vi "Open Playback Panel.vi"(9 "Offset":cluster{"dX":i32, "dY":i32}={"dX"=60, "dY"=60}, 10 "DB VI Ref":refnum<vi>, 11 "Playback in":refnum<vi>) -> (3 "Playback out":refnum<vi>)   [LabVIEW 2020]
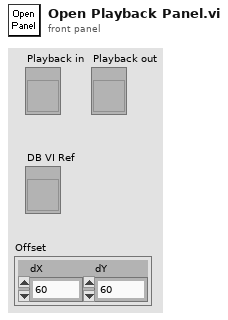
[diagram p1: front panel]
types:
  T1 = typedef "LVRectTypeDef.ctl" = cluster{"Left":i16, "Top":i16, "Right":i16, "Bottom":i16}
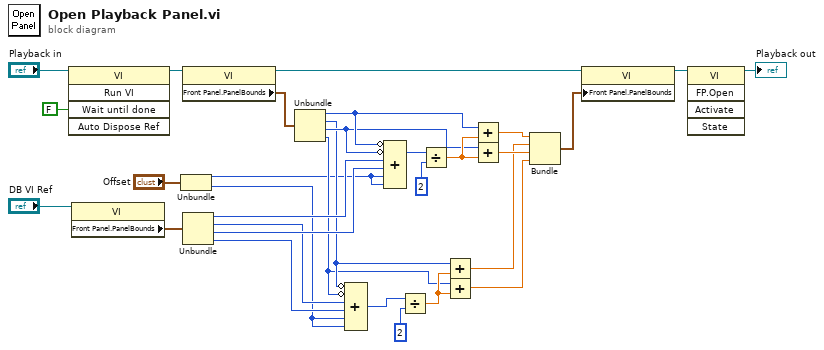
[diagram p0: block diagram]
diagram:
  n1 = invoke class="VI" method="Run VI"(reference="Playback in", "Wait until done"=FALSE ("Wait Until Done")) -> (reference out=w27:refnum<vi>)  [unwired: 3 in, 4 out]
  n2 = property class="VI"(reference="DB VI Ref") -> ("Front Panel.PanelBounds"=w24:T1)  [unwired: 1 in, 2 out]
  n3 = Unbundle("Offset") -> ("dX"=w2:i32, "dY"=w1:i32)
  n4 = property class="VI"(reference=w27) -> (reference out=w26:refnum<vi>, "Front Panel.PanelBounds"=w19:T1)  [unwired: 1 in, 1 out]
  n5 = Unbundle(w24) -> ("Left"=w23:i16, "Top"=w12:i16, "Right"=w22:i16, "Bottom"=w11:i16)
  n6 = Unbundle(w19) -> ("Left"=w14:i16, "Top"=w7:i16, "Right"=w13:i16, "Bottom"=w6:i16)
  n7 = Compound Arithmetic op=ADD(invert w7, invert w6, w12, w11, w1, w1) -> (w9:i32)
  n8 = Compound Arithmetic op=ADD(invert w14, invert w13, w23, w22, w2, w2) -> (w21:i32)
  n9 = Divide(x=w9, y=2) -> (x/y=w8:dbl)
  n10 = Divide(x=w21, y=2) -> (x/y=w15:dbl)
  n11 = Add(x=w7, y=w8) -> (x+y=w5:dbl)
  n12 = Add(x=w6, y=w8) -> (x+y=w4:dbl)
  n13 = Add(x=w14, y=w15) -> (x+y=w17:dbl)
  n14 = Add(x=w13, y=w15) -> (x+y=w16:dbl)
  n15 = Bundle(w17, w5, w16, w4) -> (w18:cluster{dbl, dbl, dbl, dbl})  [unwired: 1 in]
  n16 = property class="VI"(reference=w26, "Front Panel.PanelBounds"=w18) -> (reference out=w28:refnum<vi>)  [unwired: 1 in, 1 out]
  n17 = invoke class="VI" method="FP.Open"(reference=w28) -> (reference out=→"Playback out":refnum<vi>)  [unwired: 4 in, 4 out]
